vi "testTTL_v4.vi"() -> ()   [LabVIEW 2015]
uses:
  <vilib>/DAQmx/read.llb/DAQmx Read (Counter U32 1Chan 1Samp).vi
  <vilib>/DAQmx/write.llb/DAQmx Write (Digital Bool 1Line 1Point).vi
  <vilib>/DAQmx/write.llb/DAQmx Write (Analog Wfm 1Chan NSamp).vi
  <vilib>/DAQmx/create/channels.llb/DAQmx Create Channel (CI-Count Edges).vi
  <vilib>/DAQmx/miscellaneous.llb/DAQmx Fill In Error Info.vi
  Windows/System32/kernel32.dll
  <resource>/objmgr/daqmx.rc
panel:
  out "Counter error out":errorcluster
  out "sample count":u32
  in  "sample rate":dbl=30000.0
  in  "OEP sample clock in":tag="/Dev1/PFI1"
  in  "extra delay (ms)":dbl
  out "Curr delay (ms)":dbl(graph)
  out "max delay (ms)":dbl format="%#_10g"
  out "AO error out":errorcluster
  in  "Delay lock":bool
  out "wait time (ms)":dbl
  out "count 3":u64
  out "DO error out":errorcluster
  out "count 4":u64
  out "count 2":u64
  out "count 1":u64
  out "wait end to pulse gen end (ms)":dbl
  out "OEP to wait start (ms)":dbl caption="event rx to pulse gen start (ms)"
  out "time off (s)":dbl
  in  "Stop":bool
  out "level":sgl
  out "time on (s)":dbl
  out "New event":bool
  in  "event channel":u8=1 min=1 max=8
  out "ZMQ error out":errorcluster
  in  "port":u16=5557
  # "Timing"
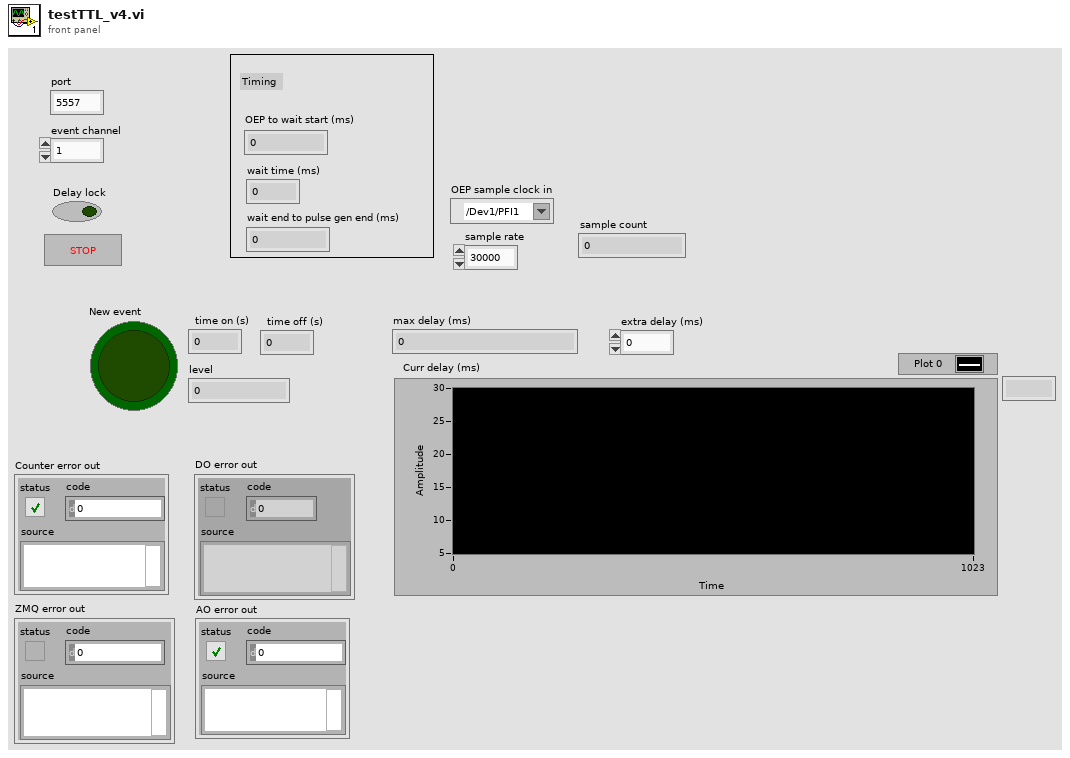
[diagram p1: front panel]
types:
  T1 = enum16{"big-endian, network order", "native, host order", "little-endian"}
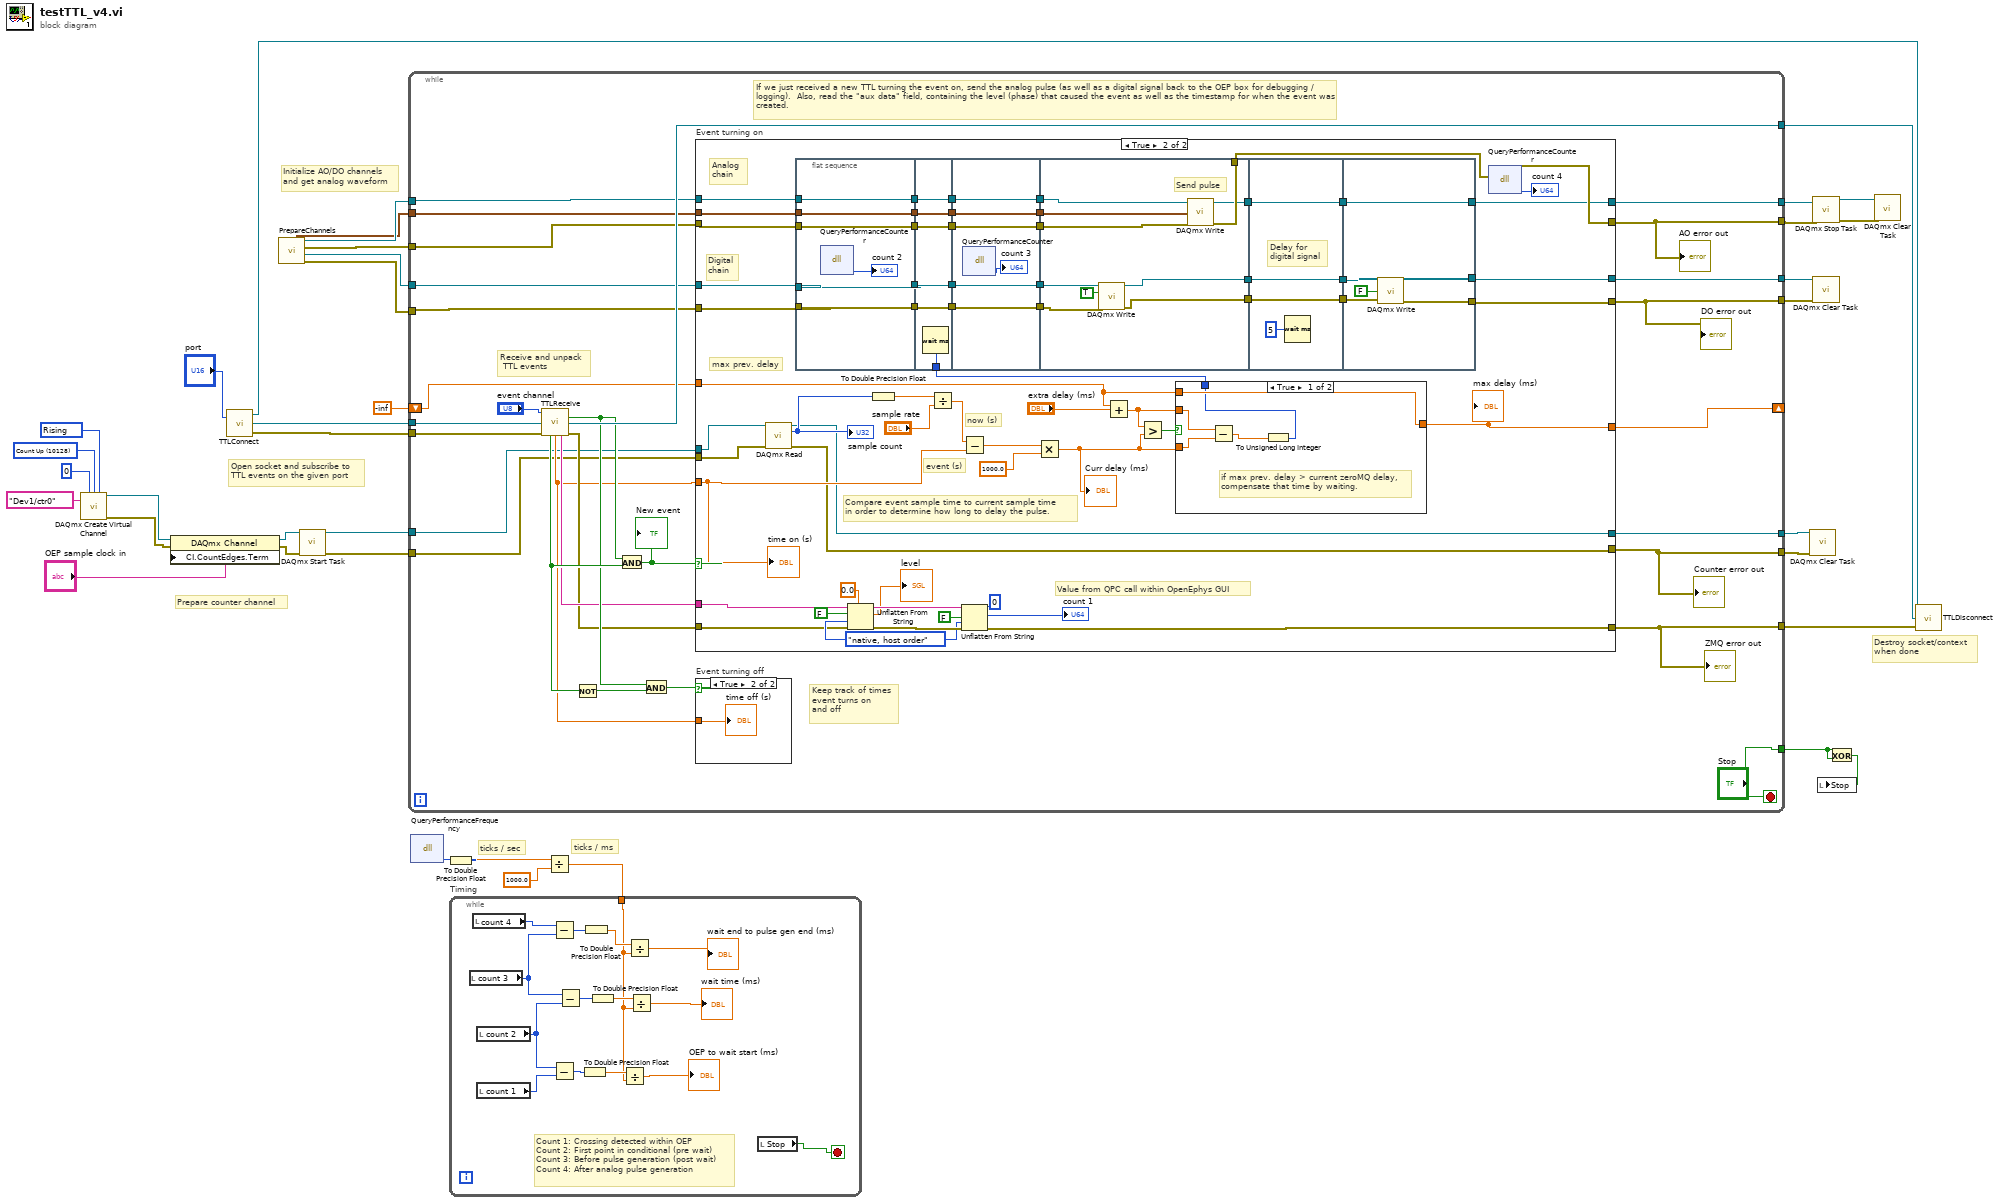
[diagram p0: block diagram]
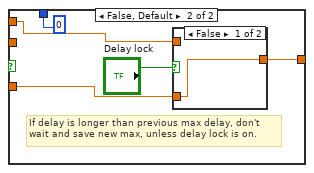
[diagram p3: hidden frame]
diagram:
  w8 = 10280 items=["Rising"=10280, "Falling"=10171] ("edge")
  w9 = 10128 items=["Count Up"=10128, "Count Down"=10124, "Externally Controlled"=10326] ("count direction")
  # "Prepare counter channel"
  # "Initialize AO/DO channels\nand get analog waveform"
  # "ticks / ms"
  # "ticks / sec"
  # "Open socket and subscribe to\nTTL events on the given port"
  # "Destroy socket/context\nwhen done"
  n1 = call-poly <vilib>:"DAQmx Create Virtual Channel.vi"("initial count"=u32 0, "count direction"=w9, "edge"=w8, "counter"=tag "Dev1/ctr0") -> ("task out"=w13:refnum<k21>, "error out"=w12:errorcluster)  [unwired: 10 in]
  n2 = property class="DAQmx Channel"(reference=w13, error in=w12, "CI.CountEdges.Term"="OEP sample clock in") -> (reference out=w7:refnum<k21>, error out=w6:errorcluster)
  n3 = call "TTLConnect.vi"("port"="port") -> ("context out"=w36:refnum<class "zmq_context.lvclass">, "socket out"=w20:refnum<class "zmq_socket.lvclass">, "error out"=w21:errorcluster)  [unwired: 1 in]
  n4 = call "PrepareChannels.vi"() -> ("DO error out"=w32:errorcluster, "DO task out"=w33:refnum<k21>, "AO error out"=w31:errorcluster, "AO task out"=w34:refnum<k21>, "Waveform Graph"=w26:waveform(dbl))  [unwired: 7 in]
  n5 = call <vilib>:"DAQmx Start Task.vi"("task/channels in"=w7, "error in"=w6) -> ("task out"=w4:refnum<k21>, "error out"=w3:errorcluster)  [unwired: 12 in]
  n6 = while {
    tunnel: w21 -> [w66]
    tunnel: [w43] -> w19
    tunnel: [w65] -> w35
    tunnel: w20 -> [w64]
    tunnel: w34 -> [w61]
    tunnel: w33 -> [w59]
    tunnel: w32 -> [w58]
    tunnel: w31 -> [w60]
    tunnel: [w48] -> w25
    tunnel: [w47] -> w24
    tunnel: [w51] -> w30
    tunnel: [w44] -> w29
    tunnel: ["Stop"] -> w28
    tunnel: w26 -> [w49]
    shift-right: [w45] -> _
    shift-left: -inf -> [w46]
    tunnel: w4 -> [w41]
    tunnel: w3 -> [w40]
    tunnel: [w39] -> w2
    tunnel: [w38] -> w1
    stop <- "Stop" stop-if-true
    # "Receive and unpack\n TTL events"
    # "If we just received a new TTL turning the event on, send the analog pulse (as well as a digital signal back to the OEP box for debugging / logging).  Also, read the \"aux data\" field, containing the level (phase) that caused the event as well as the timestamp for when the event was created."
    # "Keep track of times\nevent turns on\nand off"
    n7 = call "TTLReceive.vi"("channel"="event channel", "socket in"=w64, "error in"=w66) -> ("new TTL"=w55:bool, "socket out"=w65:refnum<class "zmq_socket.lvclass">, "event on"=w56:bool, "timestamp (s)"=w42:dbl, "aux data"=w53:string, "error out"=w52:errorcluster)  [unwired: 6 in, 1 out]
    n8 = Not(x=w56) -> (.not. x?=w57:bool)
    n9 = And(x=w55, y=w56) -> (x .and. y?=w62:bool)
    "New event" <- w62
    n10 = And(x=w55, y=w57) -> (x .and. y?=w54:bool)
    n11 = case "Event turning on" shown="True" w62 {
      tunnel: w61 -> [w74 w113]
      tunnel: w60 -> [w73 w102]
      tunnel: [w74 w111] -> w48
      tunnel: [w73 w117] -> w47
      tunnel: w59 -> [w71 w135]
      tunnel: w58 -> [w70 w118]
      tunnel: [w71 w136] -> w51
      tunnel: [w70 w122] -> w44
      tunnel: w42 -> [_ w84]
      tunnel: w53 -> [_ w127]
      tunnel: w52 -> [w72 w125]
      tunnel: [w72 w126] -> w43
      tunnel: w49 -> [_ w114]
      tunnel: w46 -> [w69 w89]
      tunnel: [w69 w120] -> w45
      tunnel: w41 -> [w68 w80]
      tunnel: w40 -> [w67 w79]
      tunnel: [w68 w77] -> w39
      tunnel: [w67 w76] -> w38
      frame False {
      }
      frame True {
        w129 = T1."native, host order" ("byte order (0:big-endian, network order)")
        # "Compare event sample time to current sample time\nin order to determine how long to delay the pulse."
        # "now (s)"
        # "event (s)"
        # "Digital\nchain"
        # "Analog \nchain"
        # "Value from QPC call within OpenEphys GUI"
        # "max prev. delay"
        n12 = call-poly <vilib>:"DAQmx Read.vi"("task/channels in"=w80, "error in"=w79) -> ("task out"=w77:refnum<k21>, "data"=w83:u32, "error out"=w76:errorcluster)  [unwired: 11 in]
        "sample count" <- w83
        n13 = flat-sequence {
          tunnel: w113 -> [w150]
          tunnel: w114 -> [w151]
          tunnel: w102 -> [w152]
          tunnel: w118 -> [w153]
          tunnel: w135 -> [w154]
          tunnel: [w154] -> w107
          tunnel: [w153] -> w106
          tunnel: [w152] -> w105
          tunnel: [w151] -> w104
          tunnel: [w150] -> w103
          tunnel: [w158] -> w101
          tunnel: [w160] -> w99
          tunnel: w119 -> [w159]
          tunnel: [w157] -> w97
          tunnel: [w156] -> w95
          tunnel: [w155] -> w93
          tunnel: w107 -> [w160]
          tunnel: w106 -> [w158]
          tunnel: w105 -> [w157]
          tunnel: w104 -> [w156]
          tunnel: w103 -> [w155]
          tunnel: w101 -> [w166]
          tunnel: [w166] -> w100
          tunnel: w99 -> [w165]
          tunnel: [w165] -> w98
          tunnel: w97 -> [w164]
          tunnel: [w164] -> w96
          tunnel: w95 -> [w163]
          tunnel: [w163] -> w94
          tunnel: w93 -> [w162]
          tunnel: [w162] -> w92
          tunnel: [w176] -> w110
          tunnel: [w175] -> w109
          tunnel: [w170] -> w108
          tunnel: [w172] -> w91
          tunnel: w92 -> [w171]
          tunnel: w94 -> [w174]
          tunnel: w96 -> [w173]
          tunnel: w98 -> [w168]
          tunnel: w100 -> [w167]
          tunnel: [w180] -> w124
          tunnel: w110 -> [w180]
          tunnel: [w179] -> w123
          tunnel: w109 -> [w179]
          tunnel: w108 -> [w177]
          tunnel: [w177] -> w112
          tunnel: [w184] -> w136
          tunnel: w124 -> [w185]
          tunnel: w123 -> [w183]
          tunnel: [w182] -> w122
          tunnel: w112 -> [w181]
          tunnel: [w181] -> w111
          frame #0 {
            n14 = dll-call lib="C:/Windows/System32/kernel32.dll" fn="QueryPerformanceCounter" label="QPC"() -> ("lpPerformanceCount"=→"count 2":u64)  [unwired: 5 in, 2 out]
          }
          frame #1 {
            n15 = Wait (ms)(milliseconds to wait=w159) -> ()  [unwired: 1 out]
          }
          frame #2 {
            n16 = dll-call lib="C:/Windows/System32/kernel32.dll" fn="QueryPerformanceCounter" label="QPC"() -> ("lpPerformanceCount"=→"count 3":u64)  [unwired: 5 in, 2 out]
          }
          frame #3 {
            # "Send pulse"
            n17 = call-poly <vilib>:"DAQmx Write.vi"("task/channels in"=w168, "data"=TRUE, "error in"=w167) -> ("task out"=w176:refnum<k21>, "error out"=w175:errorcluster)  [unwired: 10 in, 1 out]
            n18 = call-poly <vilib>:"DAQmx Write.vi"("task/channels in"=w171, "data"=w174, "error in"=w173) -> ("task out"=w170:refnum<k21>, "error out"=w172:errorcluster)  [unwired: 10 in, 1 out]
          }
          frame #4 {
            # "Delay for \ndigital signal"
            n19 = Wait (ms)(milliseconds to wait=u32 5) -> ()  [unwired: 1 out]
          }
          frame #5 {
            n20 = call-poly <vilib>:"DAQmx Write.vi"("task/channels in"=w185, "data"=FALSE, "error in"=w183) -> ("task out"=w184:refnum<k21>, "error out"=w182:errorcluster)  [unwired: 10 in, 1 out]
          }
        }
        n21 = Unflatten From String(type=sgl 0.0, binary string=w127, data includes array or string size? (T)=FALSE, byte order (0:big-endian, network order)=w129, error in (no error)=w125) -> (rest of the binary string=w131:string, value=→"level":sgl, error out=w132:errorcluster)
        n22 = To Double Precision Float(number=w83) -> (double precision float=w82:dbl)
        n23 = Divide(x=w82, y="sample rate") -> (x/y=w78:dbl)
        n24 = Unflatten From String(type=u64 0, binary string=w131, data includes array or string size? (T)=FALSE, byte order (0:big-endian, network order)=w129, error in (no error)=w132) -> (value=→"count 1":u64, error out=w126:errorcluster)  [unwired: 1 out]
        n25 = Subtract(x=w78, y=w84) -> (x-y=w86:dbl)
        n26 = Multiply(x=w86, y=1000.0 ("x")) -> (x*y=w85:dbl)
        "Curr delay (ms)" <- w85
        n27 = Add(x=w89, y="extra delay (ms)") -> (x+y=w88:dbl)
        n28 = Greater?(x=w88, y=w85) -> (0:w121:bool)
        n29 = case shown="True" w121 {
          tunnel: w85 -> [w140 w143]
          tunnel: w89 -> [w141 w144]
          tunnel: [w141 w142] -> w120
          tunnel: [w139 u32 0] -> w119
          tunnel: w88 -> [w137 _]
          frame True {
            # "if max prev. delay > current zeroMQ delay,\ncompensate that time by waiting."
            n30 = Subtract(x=w137, y=w140) -> (x-y=w138:dbl)
            n31 = To Unsigned Long Integer(number=w138) -> (unsigned 32bit integer=w139:u32)
          }
          frame False, Default {
            # "If delay is longer than previous max delay, don't\nwait and save new max, unless delay lock is on."
            n32 = case shown="False" "Delay lock" {
              tunnel: w144 -> [_ w148]
              tunnel: w143 -> [w147 _]
              tunnel: [w147 w148] -> w142
              frame False {
              }
              frame True {
              }
            }
          }
        }
        "max delay (ms)" <- w120
        n33 = dll-call lib="C:/Windows/System32/kernel32.dll" fn="QueryPerformanceCounter" label="QPC"(error in=w91) -> (error out=w117:errorcluster, "lpPerformanceCount"=→"count 4":u64)  [unwired: 4 in, 1 out]
        "time on (s)" <- w84
      }
    }
    "DO error out" <- w44
    "AO error out" <- w47
    "ZMQ error out" <- w43
    "Counter error out" <- w38
    n34 = case "Event turning off" shown="True" w54 {
      tunnel: w42 -> [_ w187]
      frame False {
      }
      frame True {
        "time off (s)" <- w187
      }
    }
  }
  n35 = dll-call lib="C:/Windows/System32/kernel32.dll" fn="QueryPerformanceFrequency"() -> ("lpFrequency"=w18:u64)  [unwired: 5 in, 2 out]
  n36 = To Double Precision Float(number=w18) -> (double precision float=w15:dbl)
  n37 = Divide(x=w15, y=1000.0) -> (x/y=w14:dbl)
  n38 = while "Timing" {
    tunnel: w14 -> [w189]
    stop <- w196 stop-if-true
    # "Count 1: Crossing detected within OEP\nCount 2: First point in conditional (pre wait)\nCount 3: Before pulse generation (post wait)\nCount 4: After analog pulse generation"
    n39 = local read "count 3"() -> (w193:u64)
    n40 = local read "count 4"() -> (w202:u64)
    n41 = local read "count 2"() -> (w192:u64)
    n42 = local read "count 1"() -> (w197:u64)
    n43 = Subtract(x=w202, y=w193) -> (x-y=w201:u64)
    n44 = Subtract(x=w192, y=w197) -> (x-y=w200:u64)
    n45 = Subtract(x=w193, y=w192) -> (x-y=w191:u64)
    n46 = To Double Precision Float(number=w200) -> (double precision float=w198:dbl)
    n47 = To Double Precision Float(number=w201) -> (double precision float=w199:dbl)
    n48 = To Double Precision Float(number=w191) -> (double precision float=w190:dbl)
    n49 = Divide(x=w198, y=w189) -> (x/y=→"OEP to wait start (ms)":dbl)
    n50 = Divide(x=w199, y=w189) -> (x/y=→"wait end to pulse gen end (ms)":dbl)
    n51 = Divide(x=w190, y=w189) -> (x/y=→"wait time (ms)":dbl)
    n52 = local read "Stop"() -> (w196:bool)
  }
  n53 = call <vilib>:"DAQmx Clear Task.vi"("task in"=w2, "error in"=w1) -> ()  [unwired: 13 in, 1 out]
  n54 = call <vilib>:"DAQmx Stop Task.vi"("task/channels in"=w25, "error in"=w24) -> ("task out"=w23:refnum<k21>, "error out"=w22:errorcluster)  [unwired: 12 in]
  n55 = call <vilib>:"DAQmx Clear Task.vi"("task in"=w30, "error in"=w29) -> ()  [unwired: 13 in, 1 out]
  n56 = Exclusive Or(1:w28, 2:w28) -> (0:w27:bool)
  n57 = local write "Stop"(w27) -> ()
  n58 = call <vilib>:"DAQmx Clear Task.vi"("task in"=w23, "error in"=w22) -> ()  [unwired: 13 in, 1 out]
  n59 = call "TTLDisconnect.vi"("error in"=w19, "socket in"=w35, "context in"=w36) -> ()  [unwired: 1 in, 1 out]
